vi "To JSON Tree.vi"(8 "error in (no error)":errorcluster, 11 "result in":refnum<class "result.lvclass">) -> (0 "error out":errorcluster, 2 "JSON Tree Out":variant, 3 "result out":refnum<class "result.lvclass">)   [LabVIEW 2015, in "result.lvclass"]
uses:
  result.lvclass
  result.lvclass/result.ctl
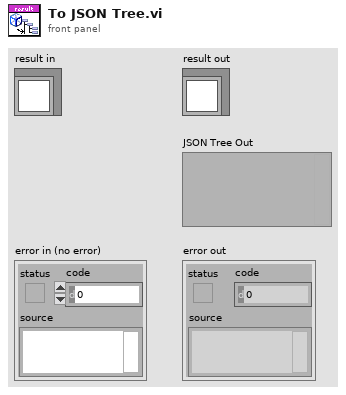
[diagram p1: front panel]
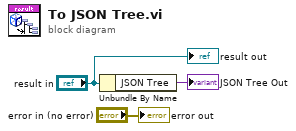
[diagram p0: block diagram]
diagram:
  n1 = Unbundle By Name("result in") -> ("JSON Tree"=→"JSON Tree Out":variant)
  "error out" <- "error in (no error)"
  "result out" <- "result in"
